vi "Iterative Minimization.vi"(9 "d rel":dbl[](array[numeric])=[10.0, 1.0, 10.0, 0.1, 1.0, 1.0, 1.0, 1.0, 1.0] format="%_4g", 10 "Array In":dbl[](array[numeric])=[7.044400000000002, 0.4286399999999992, 0.536279999999991, 1.5500139999999916, 0.17059000000000035, 0.35147, 0.30979, 0.04216999999999992, 7.418052057077897] format="%_6g") -> (1 "Minima":dbl(graph)=7.418052057077897, 2 "Array Out":dbl[](array[numeric])=[7.044400000000002, 0.4286399999999992, 0.536279999999991, 1.5500139999999916, 0.17059000000000035, 0.35147, 0.30979, 0.04216999999999992, 7.418052057077897] format="%_6g")   [LabVIEW 2016]
panel:
  in  "Abs Min":dbl=7.418052057077897
  in  "d":dbl=1e-05 format="%_4g"
  in  "Names":string[](array[string])=["Bc", "y", "mag", "theta", "v0", "v1", "g0", "width"]
  out "x = y?":bool=TRUE
  in  "# Points":i32=15
  in  "stop":bool
  in  "#Var":i32=8
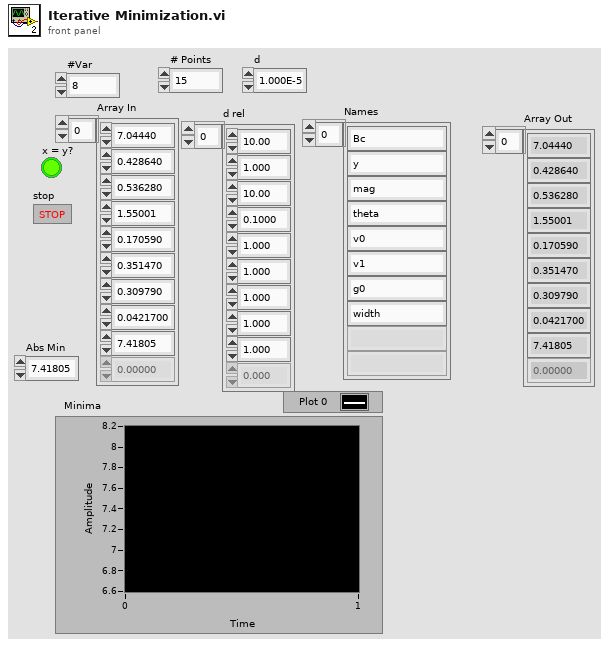
[diagram p1: front panel]
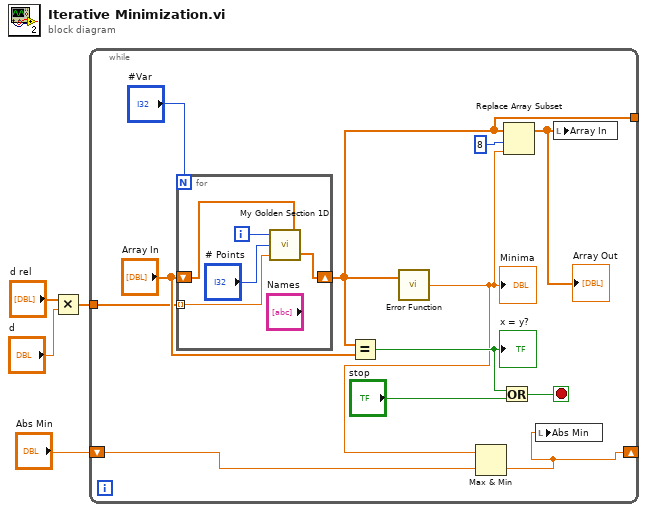
[diagram p0: block diagram]
diagram:
  n1 = Multiply(x="d rel", y="d") -> (x*y=w2:dbl[])
  n2 = while {
    tunnel: [w9] -> _
    tunnel: w2 -> [w11]
    shift-right: [w6] -> _
    shift-left: "Abs Min" -> [w7]
    stop <- w13 stop-if-true
    n3 = for {
      N: "#Var" -> [_]
      shift-right: [w19] -> w9
      shift-left: "Array In" -> [w20]
      tunnel: w11 -> [w17] mode=indexing
      i -> [w21]
      n4 = call "My Golden Section 1D.vi"("Array In"=w20, "d"=w17, "# Points"="# Points", "Var"=w21) -> ("Array Out"=w19:dbl[])
    }
    n5 = Equal?(x=w9, y="Array In") -> (x = y?=w12:bool)
    "x = y?" <- w12
    n6 = call "Error Function.vi"("Array"=w9) -> ("Error"=w8:dbl)  [unwired: 1 in]
    "Minima" <- w8
    n7 = Max & Min(x=w8, y=w7) -> (min(x,y)=w6:dbl)  [unwired: 1 out]
    n8 = Or(x=w12, y="stop") -> (x .or. y?=w13:bool)
    n9 = Replace Array Subset(array=w9, new element=w8, index=8) -> (w5:dbl[])
    "Array Out" <- w5
    n10 = local write "Abs Min"(w6) -> ()
    n11 = local write "Array In"(w5) -> ()
  }
